vi "Get Property Node.vi"(8 "error in (no error)":errorcluster) -> (0 "error out":errorcluster, 1 "Write Property out":refnum<vi>, 3 "Read Property out":refnum<vi>)   [LabVIEW 2015]
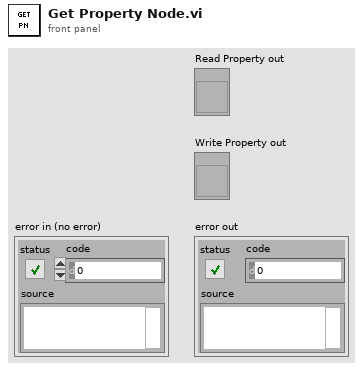
[diagram p1: front panel]
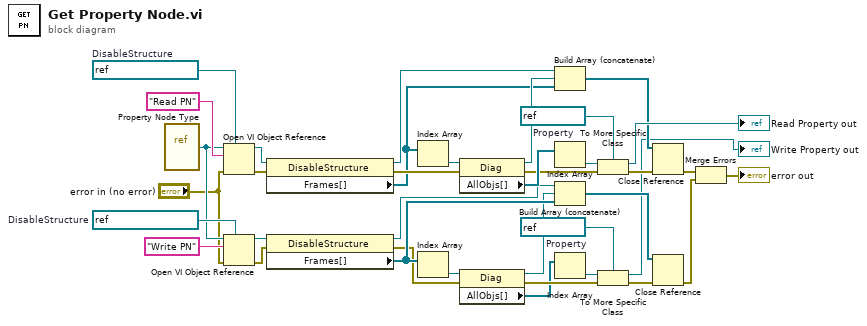
[diagram p0: block diagram]
diagram:
  w7 = refnum<vi> refnum  # Property
  w12 = refnum<vi> refnum  # DisableStructure
  w36 = refnum<vi> refnum  # Property
  w31 = refnum<vi> refnum  # DisableStructure
  n1 = vi-ref "Property Node Type.vi"() -> (w6:refnum<vi>)
  n2 = Open VI Object Reference(7:w31, 8:"error in (no error)", 10:"Read PN" ("name/order"), 11:w6) -> (0:w26:errorcluster, 3:w32:refnum<vi>)
  n3 = Open VI Object Reference(7:w12, 8:"error in (no error)", 10:"Write PN" ("name/order"), 11:w6) -> (0:w17:errorcluster, 3:w11:refnum<vi>)
  n4 = property class="DisableStructure"(reference=w32, error in=w26) -> (reference out=w22:refnum<vi>, error out=w27:errorcluster, "Frames[]"=w23:refnum<vi>[])
  n5 = property class="DisableStructure"(reference=w11, error in=w17) -> (reference out=w21:refnum<vi>, error out=w16:errorcluster, "Frames[]"=w20:refnum<vi>[])
  n6 = Index Array(array=w23) -> (element=w33:refnum<vi>)  [unwired: 1 in]
  n7 = Index Array(array=w20) -> (element=w10:refnum<vi>)  [unwired: 1 in]
  n8 = property class="Diag"(reference=w33, error in=w27) -> (reference out=w24:refnum<vi>, error out=w28:errorcluster, "AllObjs[]"=w34:refnum<vi>[])
  n9 = property class="Diag"(reference=w10, error in=w16) -> (reference out=w19:refnum<vi>, error out=w15:errorcluster, "AllObjs[]"=w9:refnum<vi>[])
  n10 = Build Array (concatenate)(w22, w24, w23) -> (w25:refnum<vi>[])
  n11 = Index Array(array=w34) -> (element=w35:refnum<vi>)  [unwired: 1 in]
  n12 = Build Array (concatenate)(w21, w19, w20) -> (w18:refnum<vi>[])
  n13 = Index Array(array=w9) -> (element=w8:refnum<vi>)  [unwired: 1 in]
  n14 = To More Specific Class(target class=w36, reference=w35, error in=w28) -> (specific class reference=→"Read Property out":refnum<vi>, error out=w29:errorcluster)
  n15 = To More Specific Class(target class=w7, reference=w8, error in=w15) -> (specific class reference=→"Write Property out":refnum<vi>, error out=w14:errorcluster)
  n16 = Close Reference(reference=w25, error in (no error)=w29) -> (error out=w3:errorcluster)
  n17 = Close Reference(reference=w18, error in (no error)=w14) -> (error out=w2:errorcluster)
  n18 = Merge Errors(w3, w2) -> (→"error out":errorcluster)
